vi "Get Default Log File Directory.vi"(8 "error in":errorcluster, 11 "Device Item Ref In":T1 format="%.0x") -> (0 "error out":errorcluster, 2 "Log File Directory String Array":string[](array[string]), 3 "Device Item Ref Out":T1 format="%.0x")   [LabVIEW 2027, in "Embedded Data Logger Scripting.lvlib"]
uses:
  Embedded Data Logger Scripting.lvlib
  <vilib>/NI VeriStand/Custom Device API/Custom Device Item Ref.ctl
  <vilib>/NI VeriStand/Custom Device API/Custom Device API.lvlib
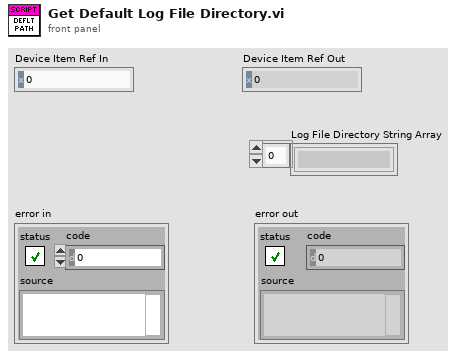
[diagram p1: front panel]
types:
  T1 = typedef "Custom Device API.lvlib/Custom Device Item Ref.ctl" = u64
  T2 = typedef "Custom Device API.lvlib/Custom Device Target Type.ctl" = enum16{"PharLap", "VxWorks", "Windows", "Linux_32_ARM", "Linux_x64"}
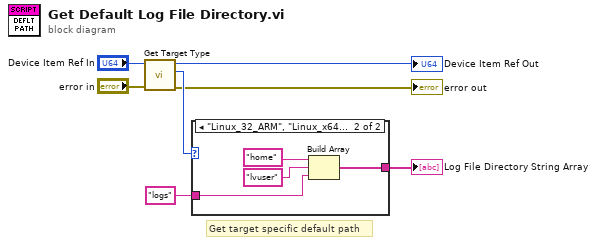
[diagram p0: block diagram]
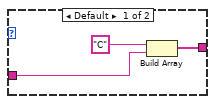
[diagram p2: hidden frame]
diagram:
  # "Get target specific default path"
  n1 = call "Get Target Type.vi"("error in"="error in", "item in"="Device Item Ref In") -> ("error out"=→"error out":errorcluster, "target type"=w5:T2, "item out"=→"Device Item Ref Out":T1)  [unwired: 7 in]
  n2 = case shown="\"Linux_32_ARM\", \"Linux_x64\"" w5 {
    tunnel: [w8 w11] -> w7
    tunnel: "logs" -> [w9 w12]
    frame Default {
      n3 = Build Array("C", w9) -> (w8:string[])
    }
    frame "Linux_32_ARM", "Linux_x64" {
      n4 = Build Array("home", "lvuser", w12) -> (w11:string[])
    }
  }
  "Log File Directory String Array" <- w7
